vi "Coin Counter.vi"() -> ()   [LabVIEW 2017]
panel:
  out "Current Width":dbl
  out "Coin":T1(ring)
  in  "Width (mm)":dbl
  out "Money ($)":dbl
  out "?":dbl(slide) scale=0.0..100.0
  # "Coin Widths:\nQuarter: 24.26\nPenny: 19.05\nDime: 17.5\nNickel: 21.21"
  # "When this says \"Loonie\",\nit means \"None\""
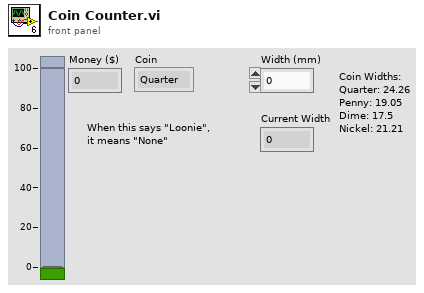
[diagram p1: front panel]
types:
  T1 = enum16{"Quarter", "Nickel", "Dime", "Penny", "Loonie", "Toonie"}
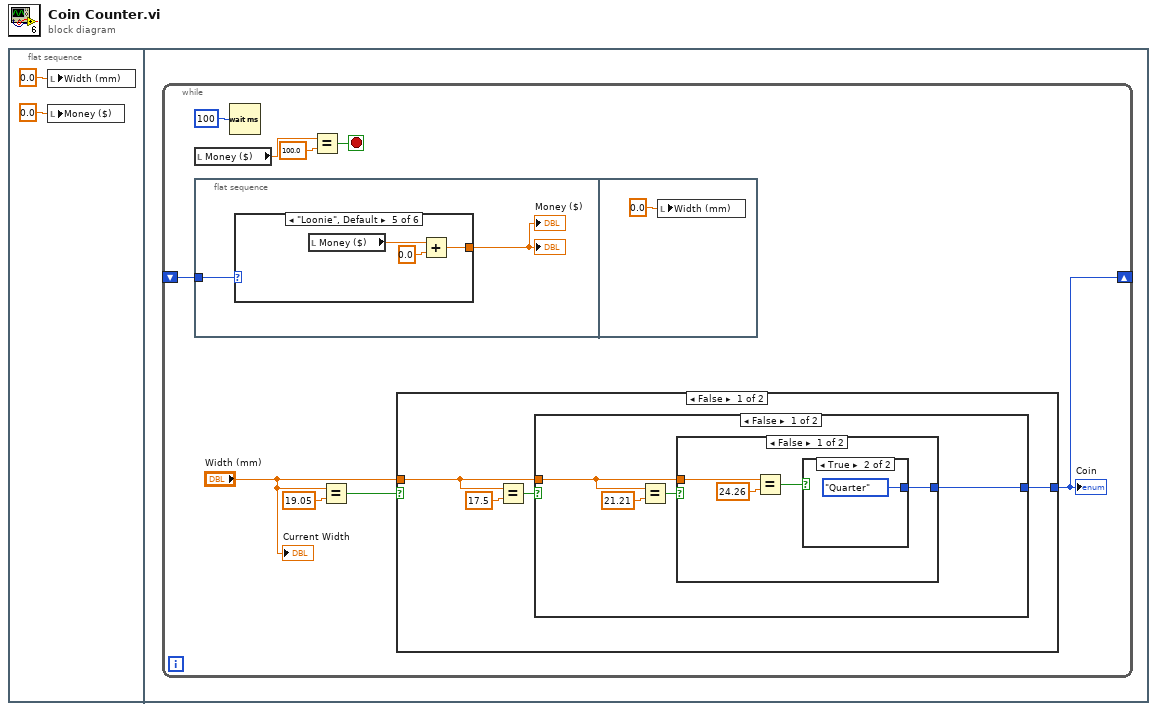
[diagram p0: block diagram]
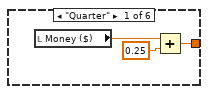
[diagram p2: hidden frame]
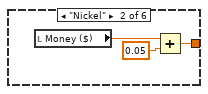
[diagram p3: hidden frame]
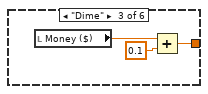
[diagram p4: hidden frame]
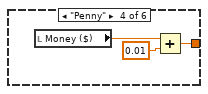
[diagram p5: hidden frame]
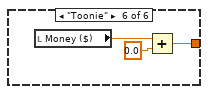
[diagram p6: hidden frame]
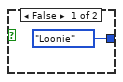
[diagram p7: hidden frame]
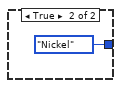
[diagram p8: hidden frame]
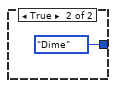
[diagram p9: hidden frame]
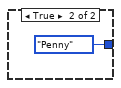
[diagram p10: hidden frame]
diagram:
  n1 = flat-sequence {
    frame #0 {
      n2 = local write "Width (mm)"(0.0 ("Width (mm)")) -> ()
      n3 = local write "Money ($)"(0.0 ("Sum")) -> ()
    }
    frame #1 {
      n4 = while {
        shift-right: [w10] -> _
        shift-left: _ -> [w11]
        stop <- w7 stop-if-true
        n5 = local read "Money ($)"() -> (w9:dbl)
        n6 = flat-sequence {
          tunnel: w11 -> [w13]
          frame #0 {
            n7 = case shown="\"Loonie\", Default" w13 {
              tunnel: [w14 w17 w20 w23 w26 w29] -> w12
              frame "Quarter" {
                n8 = local read "Money ($)"() -> (w15:dbl)
                n9 = Add(x=w15, y=0.25) -> (x+y=w14:dbl)
              }
              frame "Nickel" {
                n10 = local read "Money ($)"() -> (w19:dbl)
                n11 = Add(x=w19, y=0.05) -> (x+y=w17:dbl)
              }
              frame "Dime" {
                n12 = local read "Money ($)"() -> (w22:dbl)
                n13 = Add(x=w22, y=0.1) -> (x+y=w20:dbl)
              }
              frame "Penny" {
                n14 = local read "Money ($)"() -> (w25:dbl)
                n15 = Add(x=w25, y=0.01) -> (x+y=w23:dbl)
              }
              frame "Loonie", Default {
                n16 = local read "Money ($)"() -> (w28:dbl)
                n17 = Add(x=w28, y=0.0) -> (x+y=w26:dbl)
              }
              frame "Toonie" {
                n18 = local read "Money ($)"() -> (w31:dbl)
                n19 = Add(x=w31, y=0.0) -> (x+y=w29:dbl)
              }
            }
            "?" <- w12
            "Money ($)" <- w12
          }
          frame #1 {
            n20 = local write "Width (mm)"(0.0 ("Width (mm)")) -> ()
          }
        }
        n21 = Wait (ms)(milliseconds to wait=u32 100) -> ()  [unwired: 1 out]
        n22 = Equal?(x=w9, y=100.0) -> (x = y?=w7:bool)
        n23 = Equal?(x="Width (mm)", y=19.05) -> (x = y?=w5:bool)
        n24 = case shown="False" w5 {
          tunnel: [w33 T1."Penny" ("Coin")] -> w10
          tunnel: "Width (mm)" -> [w34 _]
          frame False {
            n25 = Equal?(x=w34, y=17.5) -> (x = y?=w35:bool)
            n26 = case shown="False" w35 {
              tunnel: [w37 T1."Dime" ("Coin")] -> w33
              tunnel: w34 -> [w38 _]
              frame False {
                n27 = Equal?(x=w38, y=21.21) -> (x = y?=w39:bool)
                n28 = case shown="False" w39 {
                  tunnel: [w41 T1."Nickel" ("Coin")] -> w37
                  tunnel: w38 -> [w43 _]
                  frame False {
                    n29 = Equal?(x=w43, y=24.26) -> (x = y?=w42:bool)
                    n30 = case shown="True" w42 {
                      tunnel: [T1."Loonie" ("Coin") T1."Quarter" ("Coin")] -> w41
                      frame False {
                      }
                      frame True {
                      }
                    }
                  }
                  frame True {
                  }
                }
              }
              frame True {
              }
            }
          }
          frame True {
          }
        }
        "Coin" <- w10
        "Current Width" <- "Width (mm)"
      }
    }
  }
